vi "Open TCP Socket.vi"(6 "local port (0)":u16, 7 "timeout ms (60000)":i32, 8 "error in (no error)":errorcluster, 9 "remote port or service name":u16, 10 "address":string, 11 "TCPSocketBasedCommHandlerBase in":refnum<class "TCPSocketBasedCommHandlerBase.lvclass">) -> (0 "error out":errorcluster, 2 "connection ID":refnum<k5>, 3 "TCPSocketBasedCommHandlerBase out":refnum<class "TCPSocketBasedCommHandlerBase.lvclass">)   [LabVIEW 2020, in "wamplv.lvlib" / "TCPSocketBasedCommHandlerBase.lvclass"]
uses:
  TCPSocketBasedCommHandlerBase.lvclass
  TCPSocketBasedCommHandlerBase.lvclass/TCPSocketBasedCommHandlerBase.ctl
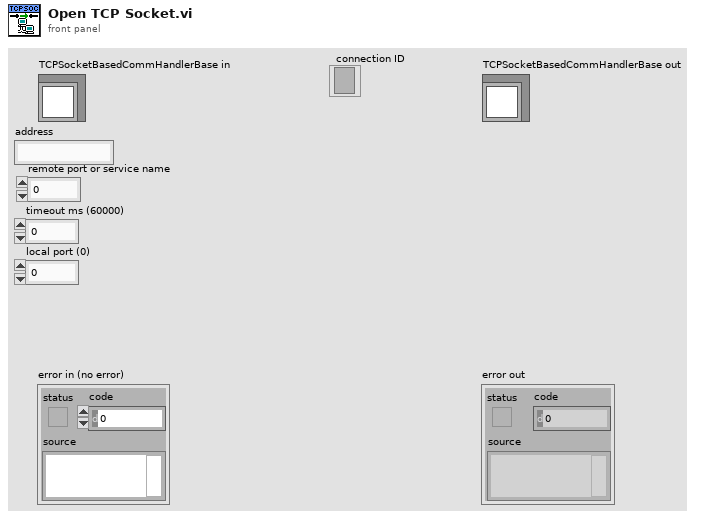
[diagram p1: front panel]
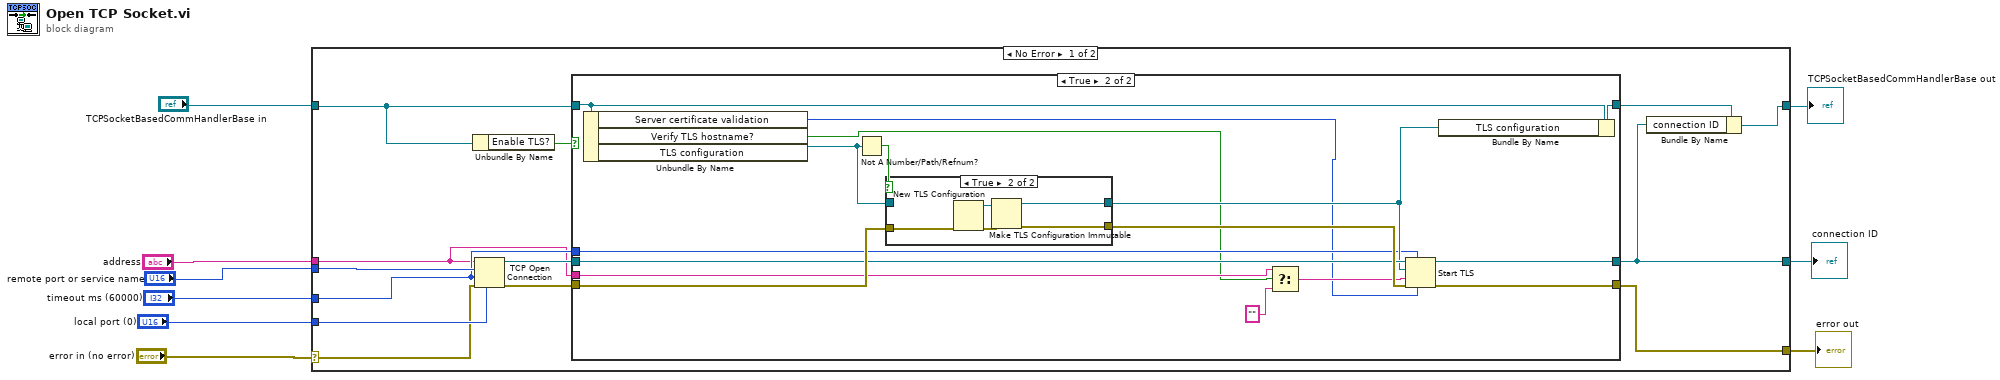
[diagram p0: block diagram]
diagram:
  n1 = case shown="No Error" "error in (no error)" {
    selector: "error in (no error)" -> [w20 w50]
    tunnel: [w12 w50] -> w8
    tunnel: [w14 w49] -> w6
    tunnel: "TCPSocketBasedCommHandlerBase in" -> [w16 w49]
    tunnel: "address" -> [w10 _]
    tunnel: "remote port or service name" -> [w22 _]
    tunnel: "timeout ms (60000)" -> [w11 _]
    tunnel: "local port (0)" -> [w21 _]
    tunnel: [w13 _] -> w1
    frame No Error {
      n2 = Unbundle By Name(w16) -> ("Enable TLS?"=w19:bool)
      n3 = TCP Open Connection(address=w10, remote port or service name=w22, timeout ms (60000)=w11, local port=w21, error in (no error)=w20) -> (connection ID=w18:refnum<k5>, error out=w17:errorcluster)
      n4 = case shown="True" w19 {
        tunnel: w18 -> [w25 w38]
        tunnel: w17 -> [w24 w40]
        tunnel: [w25 w37] -> w13
        tunnel: [w24 w36] -> w12
        tunnel: [w23 w35] -> w15
        tunnel: w16 -> [w23 w29]
        tunnel: w11 -> [_ w33]
        tunnel: w10 -> [_ w32]
        frame False {
        }
        frame True {
          n5 = Unbundle By Name(w29) -> ("Server certificate validation"=w28:enum32{"Any Trusted CA", "None"}, "Verify TLS hostname?"=w26:bool, "TLS configuration"=w27:refnum<k36>)
          n6 = Not A Number/Path/Refnum?(number/path/refnum=w27) -> (NaN/Path/Refnum?=w41:bool)
          n7 = case shown="True" w41 {
            tunnel: w27 -> [w43 _]
            tunnel: [w43 w46] -> w34
            tunnel: w40 -> [w42 w45]
            tunnel: [w42 w44] -> w39
            frame False {
            }
            frame True {
              n8 = New TLS Configuration(8:w45) -> (0:w48:errorcluster, 3:w47:refnum<k36>)  [unwired: 1 in]
              n9 = Make TLS Configuration Immutable(8:w48, 11:w47) -> (0:w44:errorcluster, 3:w46:refnum<k36>)
            }
          }
          n10 = Select(t=w32, s=w26, f="") -> (s? t:f=w31:string)
          n11 = Start TLS(6:w28, 7:w33, 8:w39, 9:w31, 10:w34, 11:w38) -> (0:w36:errorcluster, 3:w37:refnum<k5>)  [unwired: 1 out]
          n12 = Bundle By Name(cluster=w29, "TLS configuration"=w34) -> (w35:refnum<class "TCPSocketBasedCommHandlerBase.lvclass">)
        }
      }
      n13 = Bundle By Name(cluster=w15, "connection ID"=w13) -> (w14:refnum<class "TCPSocketBasedCommHandlerBase.lvclass">)
    }
    frame Error {
    }
  }
  "error out" <- w8
  "TCPSocketBasedCommHandlerBase out" <- w6
  "connection ID" <- w1
